vi "#11020_MAV_MSG_AOA_SSA.vi"(11 "mavlink_payload":u8[](array[numeric])) -> (3 "AOA_SSA":cluster{"time_usec":u64, "AOA":sgl, "SSA":sgl})   [LabVIEW 2023]
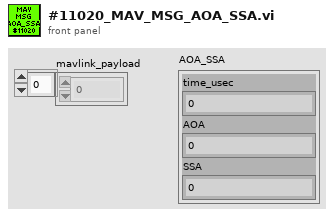
[diagram p1: front panel]
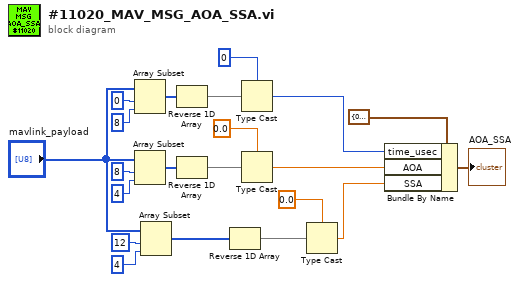
[diagram p0: block diagram]
diagram:
  n1 = Array Subset(array="mavlink_payload", index=0 ("Index"), length=8) -> (w18:u8[])
  n2 = Array Subset(array="mavlink_payload", index=8 ("Index"), length=4) -> (w12:u8[])
  n3 = Array Subset(array="mavlink_payload", index=12 ("Index"), length=4) -> (w6:u8[])
  n4 = Reverse 1D Array(array=w18) -> (reversed array=w17:u8[])
  n5 = Reverse 1D Array(array=w12) -> (reversed array=w11:u8[])
  n6 = Reverse 1D Array(array=w6) -> (reversed array=w5:u8[])
  n7 = Type Cast(type=u64 0 ("Index"), x=w17) -> (*(type *) &x=w14:u64)
  n8 = Type Cast(type=sgl 0.0 ("Index"), x=w11) -> (*(type *) &x=w8:sgl)
  n9 = Type Cast(type=sgl 0.0 ("Index"), x=w5) -> (*(type *) &x=w1:sgl)
  n10 = Bundle By Name(cluster=cluster{"time_usec":u64, "AOA":sgl, "SSA":sgl} {"time_usec"=0, "AOA"=0.0, "SSA"=0.0} ("AOA_SSA"), "time_usec"=w14, "AOA"=w8, "SSA"=w1) -> (→"AOA_SSA":cluster{"time_usec":u64, "AOA":sgl, "SSA":sgl})
